vi "data-logging-example.vi"() -> ()   [LabVIEW 2024]
uses:
  filepath-selection.ctl
panel:
  in  "Filepath Selection":T1={"Log Filepath Source"=enum."Application Relative (Auto)", "Log File Path (Manual)"=path "C:/Users/dheard/Documents/0002-labview-projects/ammonia-absorbsion-rig/data", "Log File Folder Name"="data", "log file name"="log", "Include Date in Filename"=TRUE, "Include Time in Filename"=TRUE}
  out "keep file open?":bool=TRUE
  in  "Datalogging options":T2={"Include Timestamp"=TRUE, "Include milliseconds"=FALSE, "data-precision"=3}
  out "Logged CSV out":string
  in  "format array to string":string="%.2f"
  out "array input":dbl[](array[numeric])
  out "Running":bool
  in  "CSV Data Headings":string="timestamp, data1, data2, data3, data4,"
  out "iteration":i32
  out "data4":dbl format="%.2f"
  out "data3":dbl format="%.2f"
  out "data2":dbl format="%.2f"
  out "data1":dbl format="%.2f"
  out "date string":string
  out "time string":string
  out "Log File Path":path
  out "error IO":errorcluster
  in  "Start":bool
  # "File Naming Options"
  # "Data Being Written"
  # "File Contents Options"
  # "Warning: If using mS -> Excel will not display as time format - cells can be manually changed to display correct format\nor open as text file."
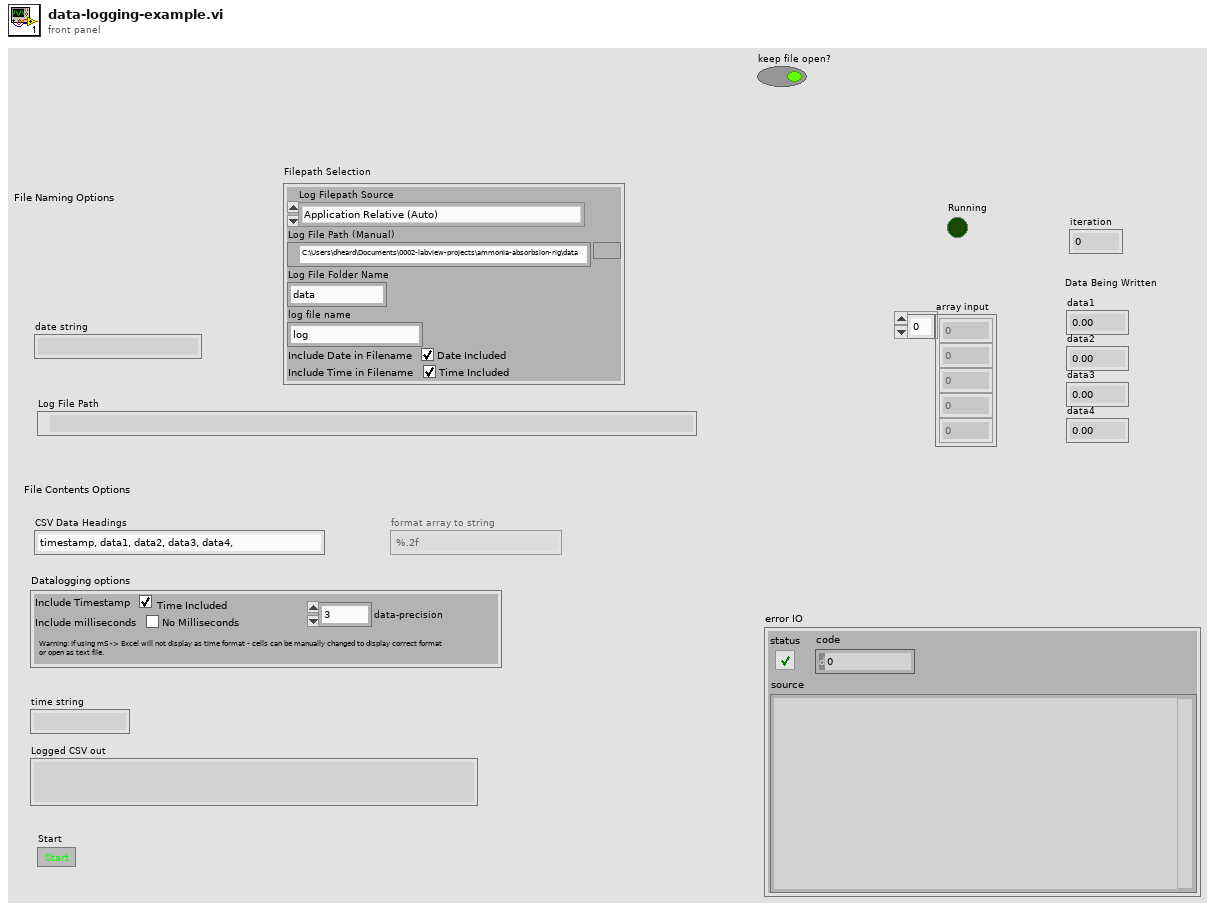
[diagram p1: front panel]
types:
  T1 = typedef "filepath-selection.ctl" = cluster{"Log Filepath Source":enum16{"Application Relative (Auto)", "VI Relative (Auto)", "Complete Path (Manual)"}, "Log File Path (Manual)":path, "Log File Folder Name":string, "log file name":string, "Include Date in Filename":bool, "Include Time in Filename":bool}
  T2 = cluster{"Include Timestamp":bool, "Include milliseconds":bool, "data-precision":i32}
  T3 = enum8{"Enabled", "Disabled", "Disabled and Grayed Out"}
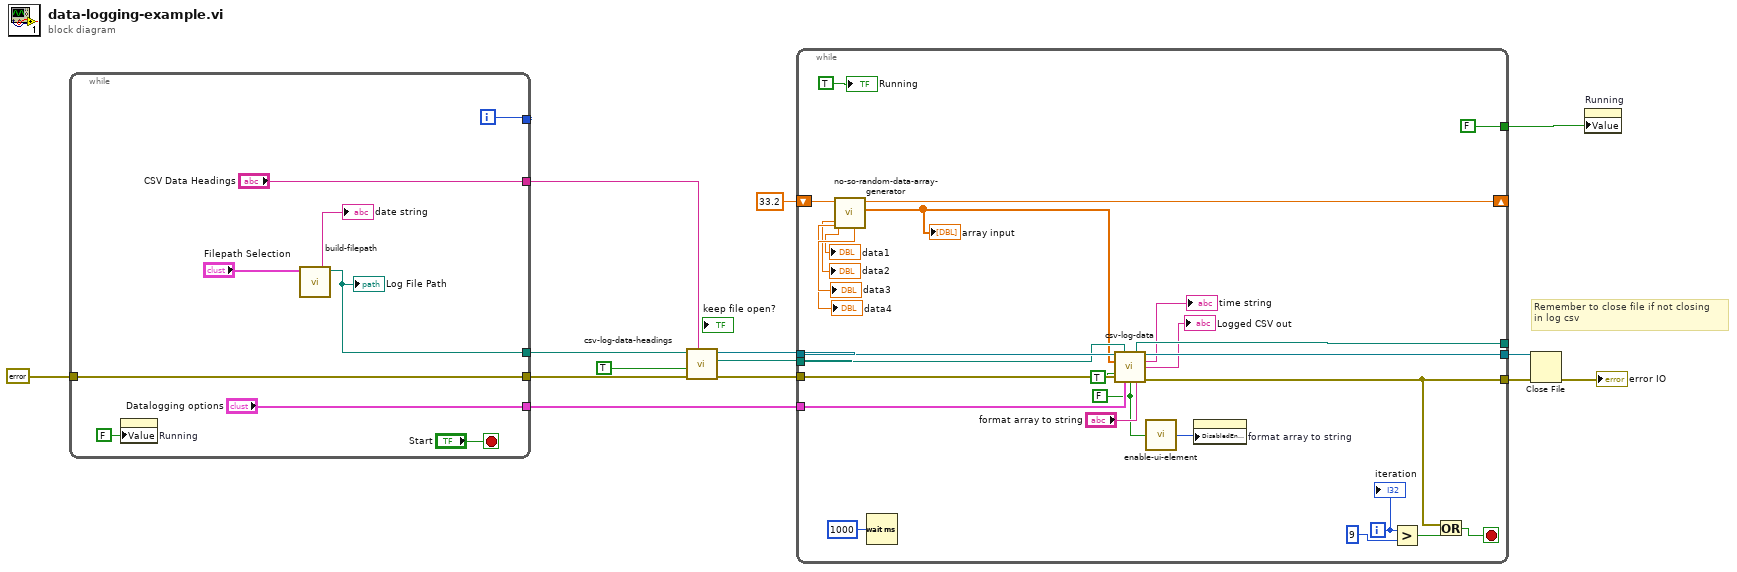
[diagram p0: block diagram]
diagram:
  # "Remember to close file if not closing\nin log csv"
  n1 = while {
    tunnel: [w22] -> w13
    tunnel: errorcluster {"status"=FALSE, "code"=0, "source"=""} ("error in") -> [w22]
    tunnel: [w21] -> _
    tunnel: [w19] -> w8
    tunnel: ["Datalogging options"] -> w6
    tunnel: ["CSV Data Headings"] -> w1
    i -> [w21]
    stop <- "Start" stop-if-true
    n2 = property on="Running" class="Bool (strict)"("Value"=FALSE ("Running")) -> ()  [unwired: 2 in, 2 out]
    n3 = call "build-filepath.vi"("Log Filepath Selection"="Filepath Selection") -> ("appended path for log file"=w19:path, "date string"=→"date string":string)  [unwired: 9 in]
    "Log File Path" <- w19
  }
  n4 = call "csv-log-data-headings.vi"("CSV Data Headings"=w1, "error in (no error)"=w13, "keep file open?"=TRUE, "Log File Path"=w8) -> ("error out"=w11:errorcluster, "Log File Path"=w5:path, "Byte Stream File out"=w12:refnum<file>)  [unwired: 5 in]
  n5 = while {
    tunnel: w12 -> [w38]
    tunnel: w11 -> [w39]
    shift-right: [w44] -> _
    shift-left: 33.2 -> [w45]
    tunnel: w6 -> [w33]
    tunnel: w5 -> [w36]
    tunnel: [w27] -> w4
    tunnel: [w37] -> w3
    tunnel: [w35] -> _
    tunnel: [FALSE ("Running")] -> w2
    i -> [w50]
    stop <- w47 stop-if-true
    w29 = FALSE ("Override Format Array?")
    n6 = call "no-so-random-data-array-generator.vi"("Numeric in"=w45) -> ("data4"=→"data4":dbl, "Array Out"=w26:dbl[], "Numeric out"=w44:dbl, "data3"=→"data3":dbl, "data2"=→"data2":dbl, "data1"=→"data1":dbl)  [unwired: 5 in]
    "array input" <- w26
    n7 = Wait (ms)(milliseconds to wait=u32 1000) -> ()  [unwired: 1 out]
    n8 = call "csv-log-data.vi"("log file Byte Stream File in"=w38, "log file path"=w36, "Data Array In"=w26, "File Open?"=TRUE, "error in (no error)"=w39, "Datalogging options"=w33, "Override Format Array?"=w29, "Format Array Override"="format array to string") -> ("log file path"=w35:path, "log file Byte Stream File out"=w37:refnum<file>, "time string"=→"time string":string, "Logged CSV out"=→"Logged CSV out":string, "error out"=w27:errorcluster)  [unwired: 3 in]
    n9 = call "enable-ui-element.vi"("Enable UI Element"=w29) -> ("UI Element State"=w28:T3)  [unwired: 8 in]
    n10 = property on="format array to string" class="Str"("DisabledEnum"=w28) -> ()  [unwired: 2 in, 2 out]
    n11 = Greater?(x=w50, y=9) -> (0:w48:bool)
    n12 = Or(x=w27, y=w48) -> (x .or. y?=w47:bool)
    "iteration" <- w50
    "Running" <- TRUE ("Running")
  }
  n13 = Close File(refnum=w3, error in=w4) -> (error out=→"error IO":errorcluster)  [unwired: 1 out]
  n14 = property on="Running" class="Bool (strict)"("Value"=w2) -> ()  [unwired: 2 in, 2 out]
